vi "Stage Position Safety.vi"(8 "error in (no error)":errorcluster, 11 "Macro Array IN":string[](array[string])) -> (0 "error out":errorcluster, 2 "Line Modified ?":bool[](array[boolean]), 3 "Modified Array OUT":string[](array[string]))   [LabVIEW 2012]
doc: "SciScan 1.2 160622"
uses:
  FGV_MacroCore_Commands.ctl
  INI/settingsIO/Settings IO_Commands.ctl
  Custom Controls and Typedefs/GFG Variable for IO.ctl
  GFG/GFG library.lvlib
panel:
  in  "OK Button":bool
  in  "Please Select your option":T1(radio)
  # "On reloading a saved macro, it is highly recommended to clear position information from commands that cause stage movement (Move.To.Pos, Z-Stack, Fast-Z).\n\nThis is a safety measure to ensure that automated movements do not cause damage to equipment or samples when sample position has changed since the macro was configured."
  # "(RECOMMENDED. Requires re-configuration of stage movement commands)"
  # "(NOT RECOMMENDED. Use at your own risk and only if you know exactly what you are doing!)"
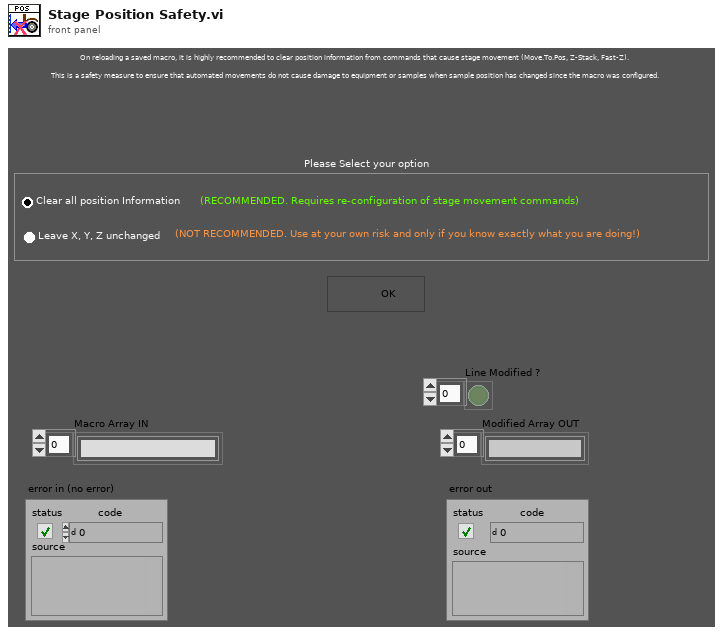
[diagram p1: front panel]
types:
  T1 = enum32{"Clear all position Information", "Leave X, Y, Z unchanged"}
  T2 = typedef "FGV_MacroCore_Commands.ctl" = enum16{"Initialize", "Get Array", "Load macro from file", "Insert Item", "Insert at End", "Edit Parameter String", "Delete instruction", "Move Items", "Save", "SaveAs", "UpdateInfoTable", "Edit Settings File", "New Macro", "Read Temp File", "Delete Multiple"}
  T3 = typedef "GFG Variable for IO.ctl" = cluster{"Variable Name":string, "Value (Variant)":variant, "data type":string}
  T4 = typedef "Settings IO_Commands.ctl" = enum16{"Write HW Settings", "Write Config Settings", "Read HW Settings", "Read Config Settings", "Write Line-Scan Settings", "Write Frame-Scan Settings", "Write Z-Stack Settings", "Read Line-Scan Settings", "Read Frame-Scan Settings", "Read Z-Stack Settings", "Read Fast-Z Settings", "Write Fast-Z Settings"}
  T5 = typedef "Macro_Action_List.ctl" = enum16{"Unknown Command", "2D.Frame.Scan", "2D.Line.Scan", "Load.Settings.File", "Move.To.Position", "Pause", "Z.Stack", "LOOP.Start", "LOOP.End", "Record", "Fast.Z", "Generic", "Slow.Z", "Tiling", "Preset.End"}
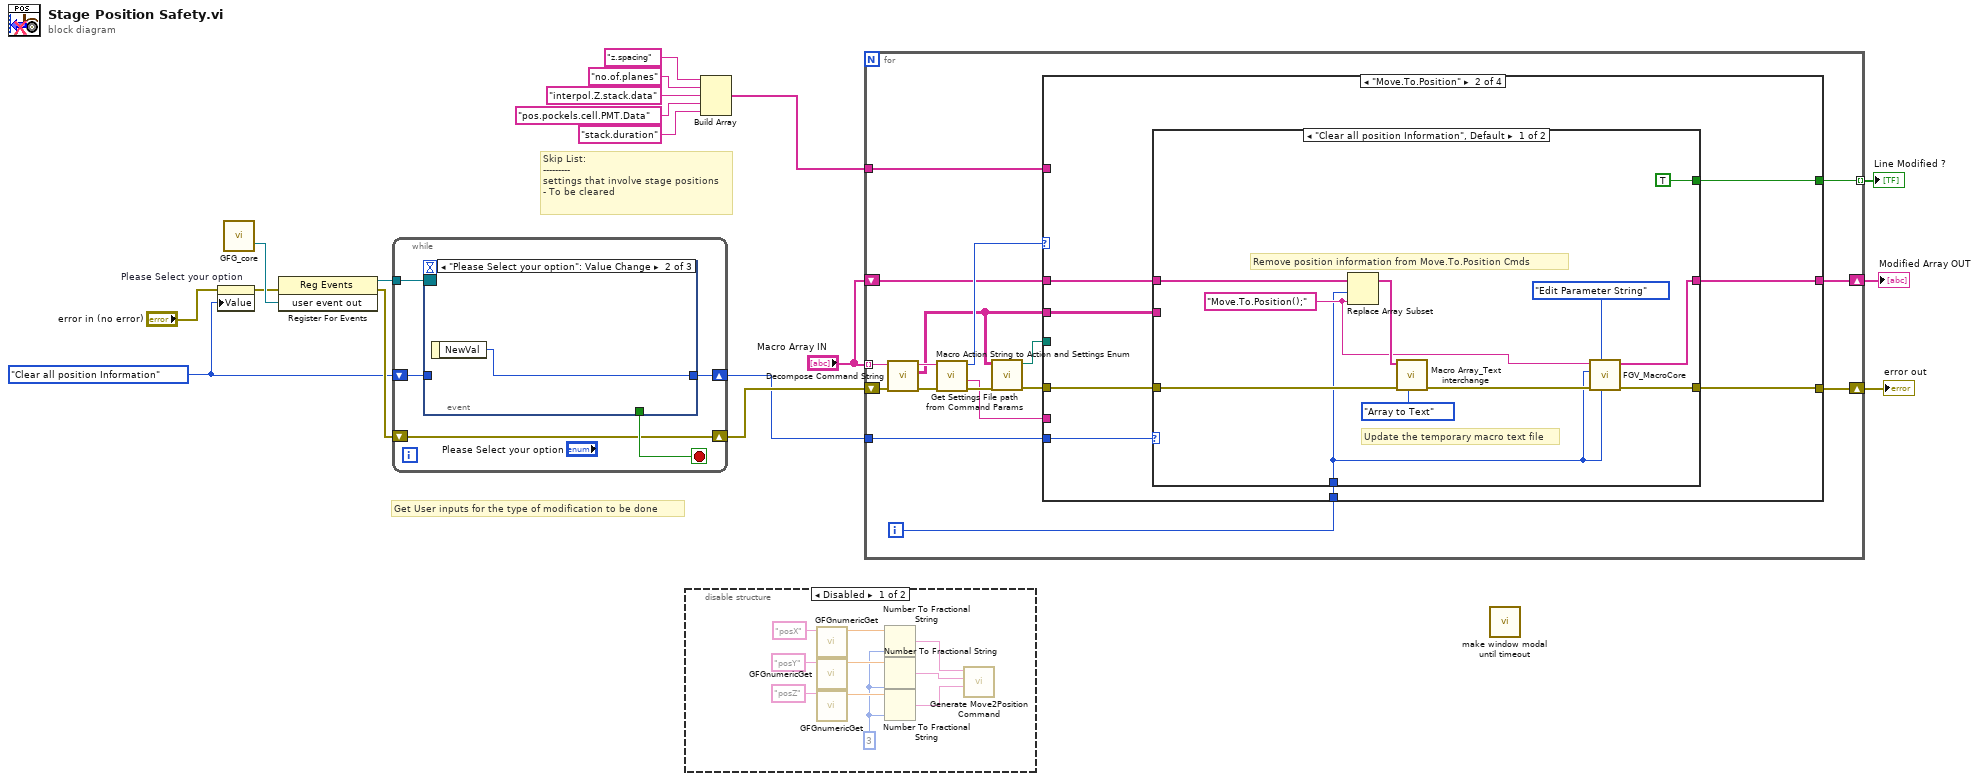
[diagram p0: block diagram]
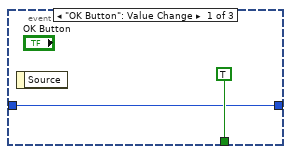
[diagram p3: hidden frame]
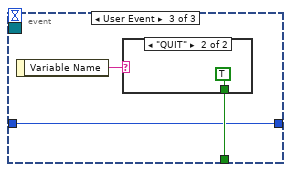
[diagram p4: hidden frame]
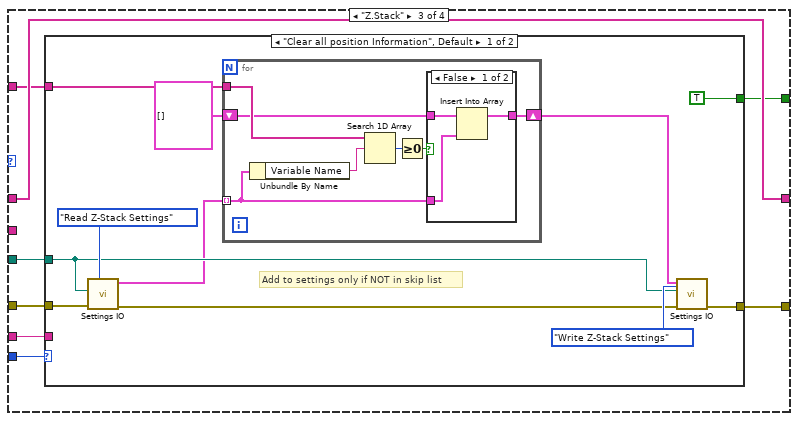
[diagram p8: hidden frame]
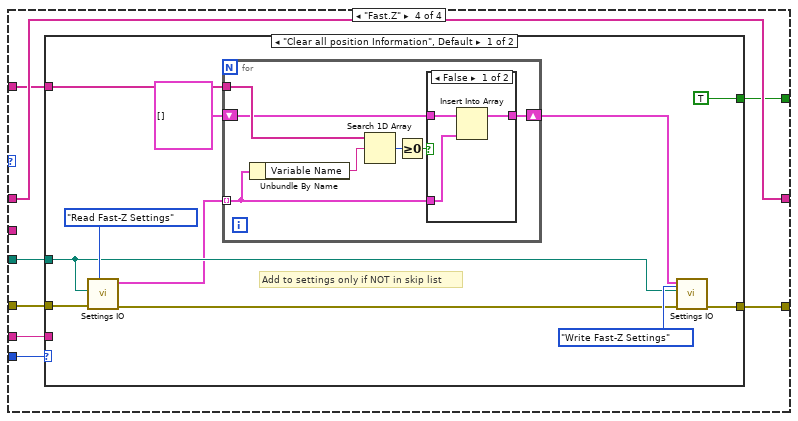
[diagram p11: hidden frame]
diagram:
  w1 = T1."Clear all position Information" ("Please Select your option")
  # "Skip List:\n---------\nsettings that involve stage positions\n- To be cleared"
  # "Get User inputs for the type of modification to be done"
  n1 = property on="Please Select your option" class="RadioBtnsControl (strict)"(error in="error in (no error)", "Value"=w1) -> (error out=w3:errorcluster)  [unwired: 1 in, 1 out]
  n2 = call "GFG_core.vi"() -> ("user event out"=w10:refnum<user-event>)  [unwired: 13 in, 6 out]
  n3 = register-events(error in=w3, w10) -> (reference out=w9:refnum<event-registration>, error out=w7:errorcluster)  [unwired: 1 in]
  n4 = while {
    tunnel: w9 -> [w23]
    shift-right: [w21] -> w6
    shift-left: w7 -> [w21]
    shift-right: [w19] -> w5
    shift-left: w1 -> [w20]
    stop <- w22 stop-if-true
    n5 = event shown="[1] \"Please Select your option\": Value Change" {
      selector: w23 -> [_ _ _]
      dyn-events: _ -> [_ _ _]
      timeout: _ -> [_ _ _]
      tunnel: [TRUE _ w28] -> w22
      tunnel: w20 -> [w24 _ w27]
      tunnel: [w24 w26 w27] -> w19
      event "OK Button": Value Change {
        n6 = event-data() -> ()  [unwired: 1 in, 1 out]
      }
      event "Please Select your option": Value Change {
        n7 = event-data() -> ("NewVal"=w26:T1)  [unwired: 1 in]
      }
      event User Event {
        n8 = event-data() -> ("Variable Name"=w29:string)  [unwired: 1 in]
        n9 = case shown="\"QUIT\"" w29 {
          tunnel: [_ TRUE] -> w28
          frame Default {
          }
          frame "QUIT" {
          }
        }
      }
    }
  }
  n10 = disable-structure shown="Disabled" {
    frame Disabled {
      w34 = i16 3 ("precision (6)")
      n11 = call "GFGnumericGet.vi"("Variable Name in"="posX") -> ("Numeric"=w35:dbl)  [unwired: 8 in, 2 out]
      n12 = call "GFGnumericGet.vi"("Variable Name in"="posY") -> ("Numeric"=w36:dbl)  [unwired: 8 in, 2 out]
      n13 = call "GFGnumericGet.vi"("Variable Name in"="posZ") -> ("Numeric"=w37:dbl)  [unwired: 8 in, 2 out]
      n14 = Number To Fractional String(number=w35, precision (6)=w34) -> (F-format string=w40:string)  [unwired: 2 in]
      n15 = Number To Fractional String(number=w36, precision (6)=w34) -> (F-format string=w39:string)  [unwired: 2 in]
      n16 = Number To Fractional String(number=w37, precision (6)=w34) -> (F-format string=w38:string)  [unwired: 2 in]
      n17 = call "Generate Move2Position Command.vi"("Pos.Z(um)"=w38, "Pos.Y(um)"=w39, "Pos.X(um)"=w40) -> ("error in (no error)"=w41:errorcluster)  [unwired: 6 in, 2 out]
    }
    frame Enabled {
    }
  }
  n18 = Build Array("z.spacing" ("Settings File Type OUT (String)"), "no.of.planes" ("Settings File Type OUT (String)"), "interpol.Z.stack.data" ("Settings File Type OUT (String)"), "pos.pockels.cell.PMT.Data" ("Settings File Type OUT (String)"), "stack.duration" ("Settings File Type OUT (String)")) -> (w12:string[])
  n19 = for {
    tunnel: "Macro Array IN" -> [w58] mode=indexing
    shift-right: [w53] -> w18
    shift-left: "Macro Array IN" -> [w54]
    tunnel: w5 -> [w51]
    tunnel: w12 -> [w45]
    shift-right: [w44] -> w11
    shift-left: w6 -> [w43]
    tunnel: [w42] -> w2 mode=indexing
    i -> [w52]
    n20 = call "Decompose Command String.vi"("Error In"=w43, "Command IN"=w58) -> ("Error Out"=w56:errorcluster, "Parameter Table"=w49:string[][], "Action"=w57:string)  [unwired: 6 in, 1 out]
    n21 = call "Macro Action String to Action and Settings Enum.vi"("error in (no error)"=w56, "Action String IN"=w57) -> ("error out"=w50:errorcluster, "Settings File Type OUT (String)"=w47:string, "Action Enum OUT"=w55:T5)  [unwired: 6 in, 1 out]
    n22 = call "Get Settings File path from Command Params.vi"("error in (no error)"=w50, "Params Array IN"=w49) -> ("error out"=w46:errorcluster, "Settings Path OUT"=w48:path)  [unwired: 8 in]
    n23 = case shown="\"Move.To.Position\"" w55 {
      tunnel: w54 -> [w60 w68 w89 w120]
      tunnel: [w60 w67 w89 w120] -> w53
      tunnel: w52 -> [_ w66 _ _]
      tunnel: w51 -> [_ w65 w83 w114]
      tunnel: w49 -> [_ w64 _ _]
      tunnel: w48 -> [_ _ w87 w118]
      tunnel: w47 -> [_ _ w88 w119]
      tunnel: w46 -> [w59 w63 w85 w116]
      tunnel: w45 -> [_ _ w86 w117]
      tunnel: [w59 w62 w84 w115] -> w44
      tunnel: [_ w61 w82 w113] -> w42
      frame Default {
      }
      frame "Move.To.Position" {
        n24 = case shown="\"Clear all position Information\", Default" w65 {
          tunnel: w68 -> [w79 w80]
          tunnel: [w75 w80] -> w67
          tunnel: w66 -> [w69 _]
          tunnel: w64 -> [_ _]
          tunnel: w63 -> [w78 w81]
          tunnel: [w77 w81] -> w62
          tunnel: [TRUE _] -> w61
          frame "Clear all position Information", Default {
            w70 = "Move.To.Position();" ("string")
            # "Remove position information from Move.To.Position Cmds"
            # "Update the temporary macro text file"
            n25 = Replace Array Subset(array=w79, new element=w70, index=w69) -> (w73:string[])
            n26 = call "Macro Array_Text interchange.vi"("Command"=enum16{"Array to Text", "Text to Array"}."Array to Text", "error in (no error)"=w78, "Macro Array IN"=w73) -> ("error out"=w71:errorcluster)  [unwired: 6 in, 2 out]
            n27 = call "FGV_MacroCore.vi"("Final Index"=w69, "MacroFGV_Commands"=FGV_MacroCore_Commands."Edit Parameter String", "Error In"=w71, "Start Index"=w69, "Macro Command or Info (String)"=w70) -> ("Error Out"=w77:errorcluster, "Macro String Array"=w75:string[])  [unwired: 2 in, 3 out]
          }
          frame "Leave X, Y, Z unchanged" {
          }
        }
      }
      frame "Z.Stack" {
        n28 = case shown="\"Clear all position Information\", Default" w83 {
          tunnel: w88 -> [_ _]
          tunnel: w87 -> [w98 _]
          tunnel: w86 -> [w94 _]
          tunnel: w85 -> [w97 w112]
          tunnel: [w96 w112] -> w84
          tunnel: [TRUE _] -> w82
          frame "Clear all position Information", Default {
            # "Add to settings only if NOT in skip list"
            n29 = call "Settings IO.vi"("SettingsFileIO_Commands"=Settings_IO_Commands."Read Z-Stack Settings", "Error In"=w97, "File Path (for scan specific settings)"=w98) -> ("Error Out"=w91:errorcluster, "Settings Array OUT"=w95:T3[])  [unwired: 6 in, 1 out]
            n30 = for {
              tunnel: w95 -> [w101] mode=indexing
              tunnel: w94 -> [w106]
              shift-right: [w102] -> w92
              shift-left: T3[] [] -> [w103]
              n31 = Unbundle By Name(w101) -> ("Variable Name"=w107:string)
              n32 = Search 1D Array(1D array=w106, element=w107) -> (index of element=w105:i32)  [unwired: 1 in]
              n33 = Greater Or Equal To 0?(x=w105) -> (x >= 0?=w104:bool)
              n34 = case shown="False" w104 {
                tunnel: w103 -> [w110 w111]
                tunnel: [w109 w111] -> w102
                tunnel: w101 -> [w108 _]
                frame False {
                  n35 = Insert Into Array(array=w110, new element=w108) -> (w109:T3[])  [unwired: 1 in]
                }
                frame True {
                }
              }
            }
            n36 = call "Settings IO.vi"("SettingsFileIO_Commands"=Settings_IO_Commands."Write Z-Stack Settings", "Error In"=w91, "File Path (for scan specific settings)"=w98, "Settings Array IN"=w92) -> ("Error Out"=w96:errorcluster)  [unwired: 5 in, 2 out]
          }
          frame "Leave X, Y, Z unchanged" {
          }
        }
      }
      frame "Fast.Z" {
        n37 = case shown="\"Clear all position Information\", Default" w114 {
          tunnel: w119 -> [_ _]
          tunnel: w118 -> [w129 _]
          tunnel: w117 -> [w125 _]
          tunnel: w116 -> [w128 w143]
          tunnel: [w127 w143] -> w115
          tunnel: [TRUE _] -> w113
          frame "Clear all position Information", Default {
            # "Add to settings only if NOT in skip list"
            n38 = call "Settings IO.vi"("SettingsFileIO_Commands"=Settings_IO_Commands."Read Fast-Z Settings", "Error In"=w128, "File Path (for scan specific settings)"=w129) -> ("Error Out"=w122:errorcluster, "Settings Array OUT"=w126:T3[])  [unwired: 6 in, 1 out]
            n39 = for {
              tunnel: w126 -> [w132] mode=indexing
              tunnel: w125 -> [w137]
              shift-right: [w133] -> w123
              shift-left: T3[] [] -> [w134]
              n40 = Unbundle By Name(w132) -> ("Variable Name"=w138:string)
              n41 = Search 1D Array(1D array=w137, element=w138) -> (index of element=w136:i32)  [unwired: 1 in]
              n42 = Greater Or Equal To 0?(x=w136) -> (x >= 0?=w135:bool)
              n43 = case shown="False" w135 {
                tunnel: w134 -> [w141 w142]
                tunnel: [w140 w142] -> w133
                tunnel: w132 -> [w139 _]
                frame False {
                  n44 = Insert Into Array(array=w141, new element=w139) -> (w140:T3[])  [unwired: 1 in]
                }
                frame True {
                }
              }
            }
            n45 = call "Settings IO.vi"("SettingsFileIO_Commands"=Settings_IO_Commands."Write Fast-Z Settings", "Error In"=w122, "File Path (for scan specific settings)"=w129, "Settings Array IN"=w123) -> ("Error Out"=w127:errorcluster)  [unwired: 5 in, 2 out]
          }
          frame "Leave X, Y, Z unchanged" {
          }
        }
      }
    }
  }
  "error out" <- w11
  "Modified Array OUT" <- w18
  "Line Modified ?" <- w2
  n46 = call "make window modal until timeout.vi"() -> ()  [unwired: 12 in]
